vi "Close.vi"(8 "error in":errorcluster, 11 "Error in":refnum<class "Error.lvclass">) -> (0 "error out":errorcluster, 3 "Error out":refnum<class "Error.lvclass">)   [LabVIEW 2023, in "Error.lvclass"]
uses:
  Error.lvclass
  Error.lvclass/Error.ctl
  <vilib>/ADAS Replay HIL/AdasHilServices/AdasHilServices Fill In Error Info Ex.vi
  <vilib>/ADAS Replay HIL/AdasHilServices/AdasHilChannelServices.lvlib
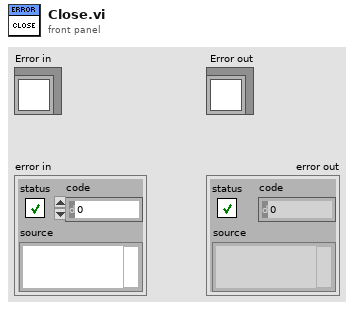
[diagram p1: front panel]
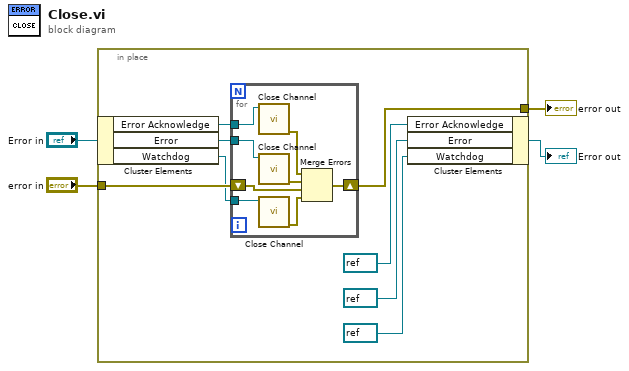
[diagram p0: block diagram]
diagram:
  n1 = in-place {
    in-place-border: "error in" -> [w12]
    in-place-border: [w11] -> w3
    n2 = in-place-cluster #1("Error in") -> ("Error Acknowledge"=w10:refnum<k21>, "Error"=w9:refnum<k21>, "Watchdog"=w7:refnum<k21>)
    n3 = for {
      tunnel: w10 -> [w20]
      tunnel: w9 -> [w19]
      shift-right: [w18] -> w11
      shift-left: w12 -> [w15]
      tunnel: w7 -> [w14]
      n4 = call <vilib>:"Close Channel.vi"("ADAS HIL Channel"=w20) -> ("error out"=w17:errorcluster)  [unwired: 10 in]
      n5 = call <vilib>:"Close Channel.vi"("ADAS HIL Channel"=w19) -> ("error out"=w16:errorcluster)  [unwired: 10 in]
      n6 = call <vilib>:"Close Channel.vi"("ADAS HIL Channel"=w14) -> ("error out"=w13:errorcluster)  [unwired: 10 in]
      n7 = Merge Errors(w17, w16, w15, w13) -> (w18:errorcluster)
    }
    n8 = in-place-cluster #1("Error Acknowledge"=refnum<k21> refnum, "Error"=refnum<k21> refnum, "Watchdog"=refnum<k21> refnum) -> (→"Error out":refnum<class "Error.lvclass">)
  }
  "error out" <- w3
